vi "Edit_meas_setup_file.vi"(0 "Comments":string, 4 "Sampling rate":dbl, 5 "Sampling time (s)":dbl format="%.2f", 6 "No of blocks":i32, 7 "Meas setup file":string="Colourimeter setup") -> ()   [LabVIEW 2010]
uses:
  Globals/Constants_global.vi
panel:
  out "Appended string":string
  out "Output string":string
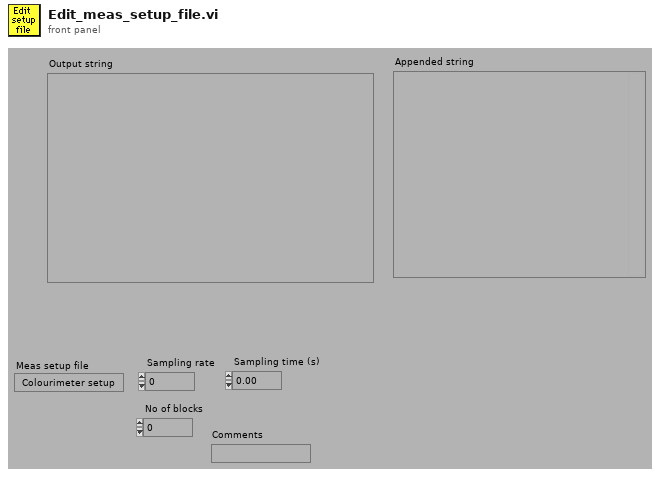
[diagram p1: front panel]
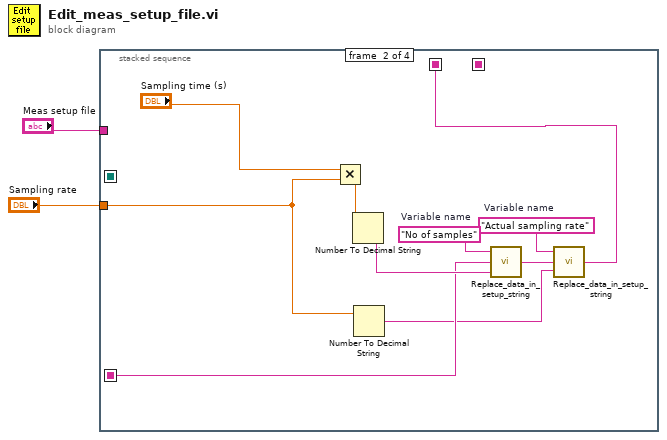
[diagram p0: block diagram]
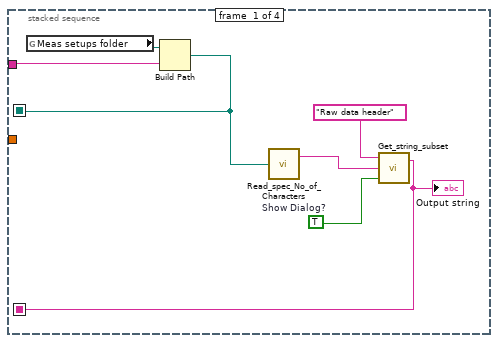
[diagram p2: hidden frame]
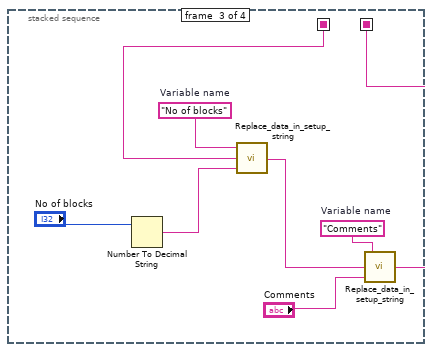
[diagram p3: hidden frame]
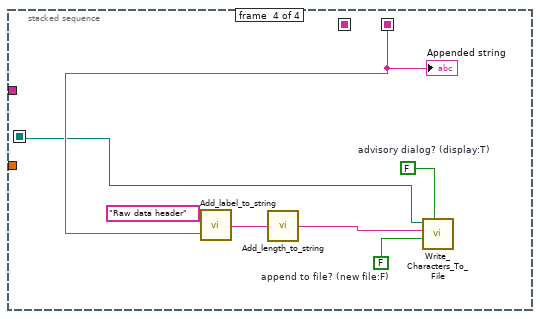
[diagram p4: hidden frame]
diagram:
  n1 = stacked-sequence {
    seq-local: [w8 _ _ _] -> [_ w15 _ _]
    seq-local: [_ w11 _ _] -> [_ _ w26 _]
    seq-local: [_ _ w21 _] -> [_ _ _ w30]
    seq-local: [w4 _ _ _] -> [_ _ _ w28]
    tunnel: "Meas setup file" -> [w5 _ _ _]
    tunnel: "Sampling rate" -> [_ w10 _ _]
    frame #0 {
      w3 = TRUE  # Show Dialog?
      n2 = global read "Constants_global.vi" "Meas setups folder"() -> (w6:path)
      n3 = Build Path(base path=w6, name or relative path=w5) -> (appended path=w4:path)
      n4 = call "Read_spec_No_of_Characters.vi"("Filename"=w4) -> ("character string"=w7:string)  [unwired: 1 out]
      n5 = call "Get_string_subset.vi"("Show Dialog?"=w3, "String to split"=w7, "File Label"="Raw data header") -> ("Output string"=w8:string)  [unwired: 1 out]
      "Output string" <- w8
    }
    frame #1 {
      w13 = "Actual sampling rate"  # Variable name
      w17 = "No of samples"  # Variable name
      n6 = Multiply(x="Sampling time (s)", y=w10) -> (x*y=w19:dbl)
      n7 = Number To Decimal String(number=w19) -> (decimal integer string=w18:string)  [unwired: 1 out]
      n8 = Number To Decimal String(number=w10) -> (decimal integer string=w12:string)  [unwired: 1 out]
      n9 = call "Replace_data_in_setup_string.vi"("New data string"=w18, "Input string"=w15, "Variable name"=w17) -> ("Appended string"=w14:string)
      n10 = call "Replace_data_in_setup_string.vi"("New data string"=w12, "Input string"=w14, "Variable name"=w13) -> ("Appended string"=w11:string)
    }
    frame #2 {
      w23 = "Comments"  # Variable name
      w27 = "No of blocks"  # Variable name
      n11 = Number To Decimal String(number="No of blocks") -> (decimal integer string=w24:string)  [unwired: 1 out]
      n12 = call "Replace_data_in_setup_string.vi"("New data string"=w24, "Input string"=w26, "Variable name"=w27) -> ("Appended string"=w22:string)
      n13 = call "Replace_data_in_setup_string.vi"("New data string"="Comments", "Input string"=w22, "Variable name"=w23) -> ("Appended string"=w21:string)
    }
    frame #3 {
      w33 = FALSE  # advisory dialog? (display:T)
      w34 = FALSE  # append to file? (new file:F)
      n14 = call "Add_label_to_string.vi"("String to write"=w30, "File Label"="Raw data header") -> ("Output string"=w31:string)
      n15 = call "Add_length_to_string.vi"("String in"=w31) -> ("String out"=w29:string)
      n16 = call "Write_Characters_To_File.vi"("file path (dialog if empty)"=w28, "advisory dialog? (display:T)"=w33, "character string"=w29, "append to file? (new file:F)"=w34) -> ()  [unwired: 1 in, 4 out]
      "Appended string" <- w30
    }
  }
